vi "PI_GCS3_Sample_Application_Fault_Reaction.vi"() -> ()   [LabVIEW 2026]
doc: "This VI demonstrates how to reset a PI GCS3 system from fault axis state. The diagram shows how to combine the driver VIs for these tasks.\n\nWarning: Before running this VI, modify the interface settings on the block diagram to reflect your configuration. The predefined settings provided with the VI probably do not match your system.\n\nCompatibility: This sample requires a PI GCS 3.0 controller."
uses:
  Low Level/SpecialCommand/ModeOfOperation.ctl
  Low Level/Communication/Interface Settings.ctl
  Low Level/GeneralCommands/ParameterInfoSet.ctl
  Low Level/GeneralCommands/Status.ctl
panel:
  out "Original PID values":string[](array[string])
  out "Restored Status of motion group":T1[](array[typedef])
  out "Fault Status":T1[](array[typedef])
  out "Initial Status":T1[](array[typedef])
  out "Axis Parameter Configuration":T2[](array[typedef])
  out "error out":errorcluster
  in  "error in":errorcluster
  in  "stop":bool
  out "Identification":string
  # "This VI demonstrates how to reset a PI GCS3 system from fault axis state.\nThe diagram shows how to combine the driver VIs for these tasks. \n\nWarning: Before running this VI, modify the interface settings on the block diagram to reflect your configuration.\n                 The predefined settings provided with the VI probably do not match your system.\n\nCompatibility: This sample requires a PI GCS 3.0 controller."
  # "Error"
  # "Referenced?"
  # "Closed Loop"
  # "Axis enabled?"
  # "On target?"
  # "Fault Reaction Active?"
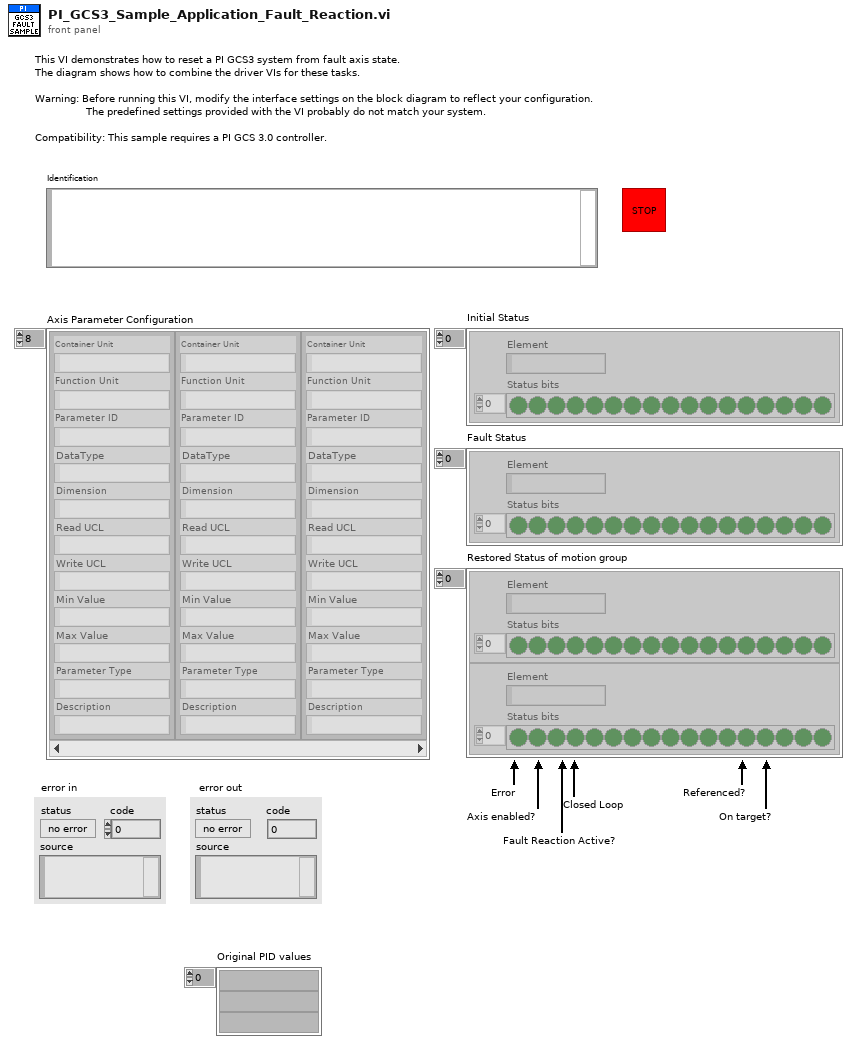
[diagram p1: front panel]
types:
  T1 = typedef "Status.ctl" = cluster{"Element":string, "Status bits":bool[]}
  T2 = typedef "ParameterInfoSet.ctl" = cluster{"Container Unit":string, "Function Unit":string, "Parameter ID":string, "DataType":string, "Dimension":string, "Read UCL":string, "Write UCL":string, "Min Value":string, "Max Value":string, "Parameter Type":string, "Description":string}
  T3 = typedef "Interface Settings.ctl" = cluster{"Interface":u16, "Timeout":u32, "RS232 settings":cluster{"Portnumber":u8, "Baudrate":u16}, "TCP/IP settings":cluster{"Host address/name":string, "Port":i32, "Board":i32, "TCP/IP Search?":bool}, "USB settings":cluster{"S/N":string, "USB Search?":bool}, "DaisyChain settings":cluster{"Register DC":bool, "DaisyChain Search?":bool, "Device ID":i32}, "DLL for Device":u16}
  T4 = typedef "ModeOfOperation.ctl" = enum16{"Open", "Open-Loop Position", "Closed-Loop Position", "Open-Loop Velocity", "Closed-Loop Velocity", "Open-Loop Force", "Closed-Loop Force", "Step Operation"}
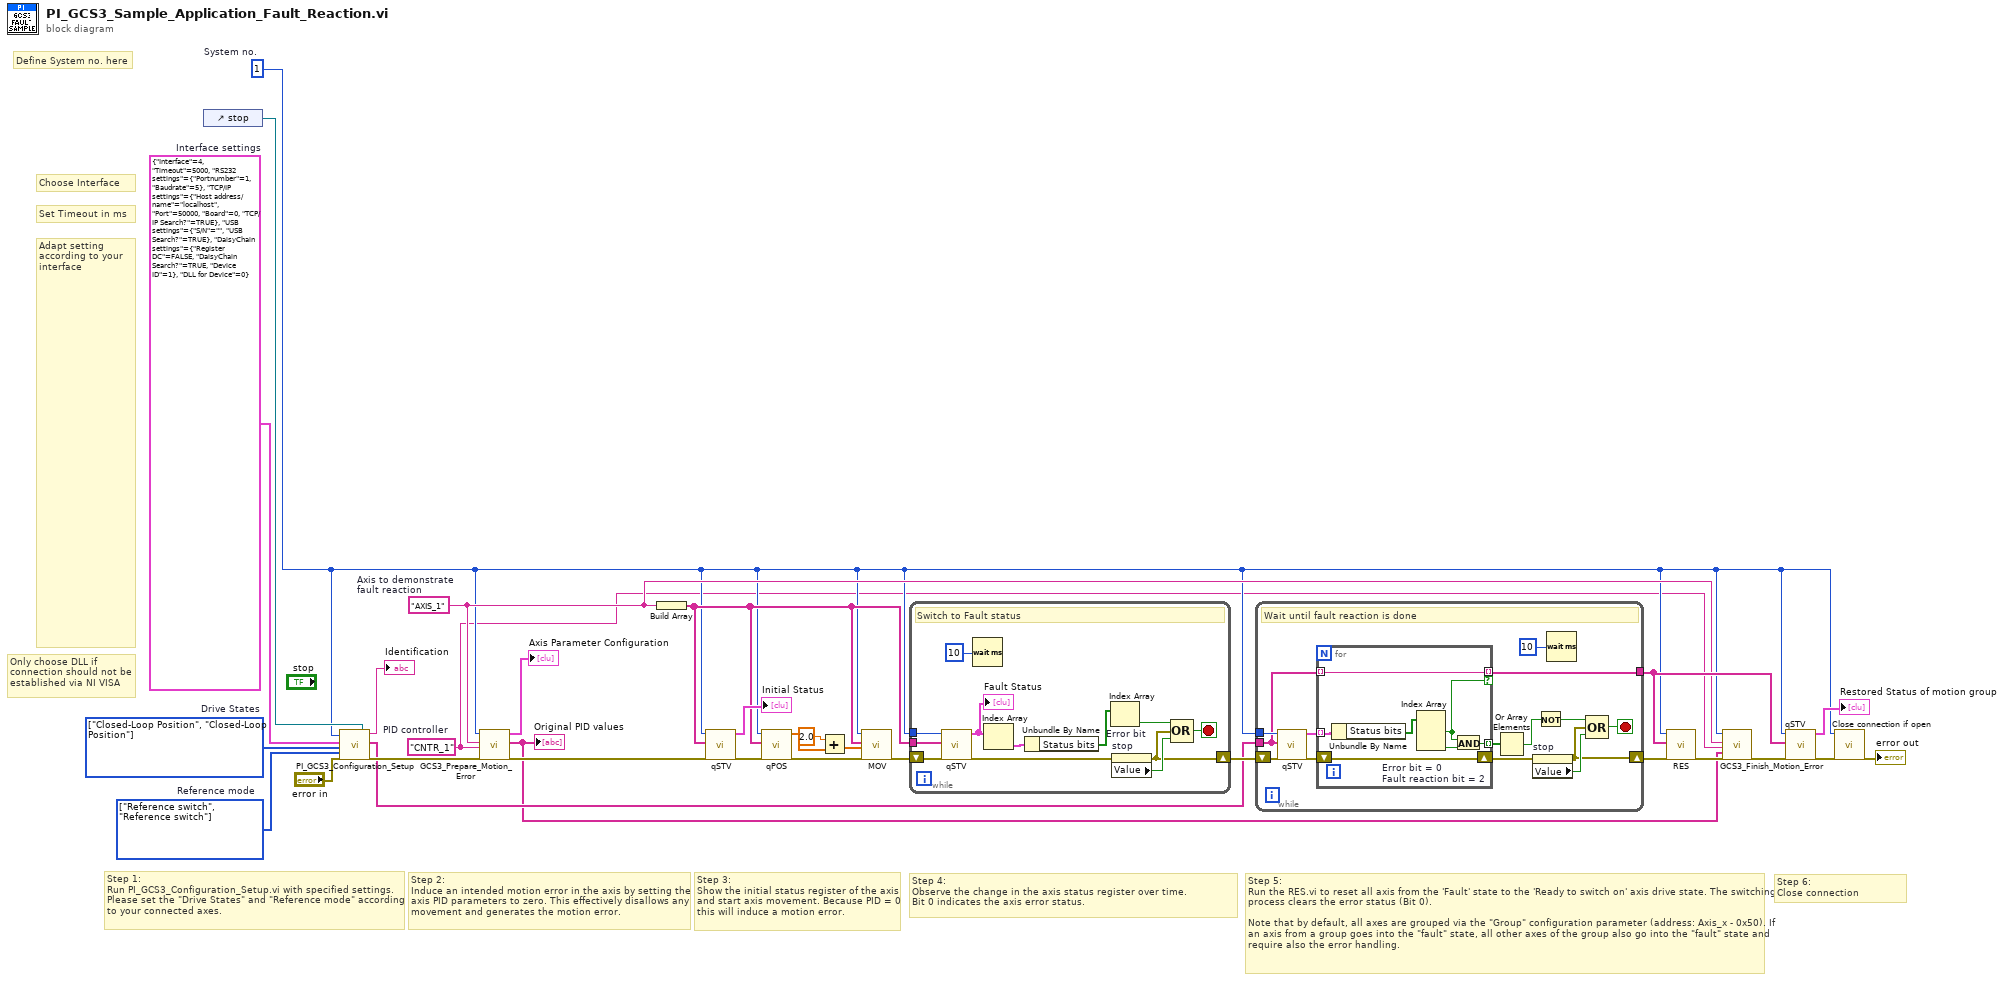
[diagram p0: block diagram]
diagram:
  w8 = T3 {"Interface"=4, "Timeout"=5000, "RS232 settings"={"Portnumber"=1, "Baudrate"=5}, "TCP/IP settings"={"Host address/name"="localhost", "Port"=50000, "Board"=0, "TCP/IP Search?"=TRUE}, "USB settings"={"S/N"="", "USB Search?"=TRUE}, "DaisyChain settings"={"Register DC"=FALSE, "DaisyChain Search?"=TRUE, "Device ID"=1}, "DLL for Device"=0}  # Interface settings
  w2 = "CNTR_1"  # PID controller
  w4 = "AXIS_1"  # Axis to demonstrate fault reaction
  w28 = T4[] [enum."Closed-Loop Position", enum."Closed-Loop Position"] items=["Open", "Open-Loop Position", "Closed-Loop Position", "Open-Loop Velocity", "Closed-Loop Velocity", "Open-Loop Force", "Closed-Loop Force", "Step Operation"]  # Drive States
  w29 = enum16{"Do not reference", "Reference switch"}[] [enum."Reference switch", enum."Reference switch"] items=["Do not reference", "Reference switch"]  # Reference mode
  w3 = 1  # System no.
  # "Define System no. here"
  # "Adapt setting according to your interface"
  # "Set Timeout in ms"
  # "Choose Interface"
  # "Only choose DLL if connection should not be established via NI VISA"
  # "Step 5:\nRun the RES.vi to reset all axis from the 'Fault' state to the 'Ready to switch on' axis drive state. The switching process clears the error status (Bit 0).\n\nNote that by default, all axes are grouped via the \"Group\" configuration parameter (address: Axis_x - 0x50). If an axis from a group goes into the \"fault\" state, all other axes of the group also go into the \"fault\" state and require also the error handling."
  # "Step 4:\nObserve the change in the axis status register over time.\nBit 0 indicates the axis error status."
  # "Step 3:\nShow the initial status register of the axis\nand start axis movement. Because PID = 0\nthis will induce a motion error."
  # "Step 2:\nInduce an intended motion error in the axis by setting the\naxis PID parameters to zero. This effectively disallows any movement and generates the motion error."
  # "Step 6:\nClose connection"
  # "Step 1:\nRun PI_GCS3_Configuration_Setup.vi with specified settings.\nPlease set the \"Drive States\" and \"Reference mode\" according\nto your connected axes."
  n1 = control-ref of="stop"() -> (w26:refnum<vi>)
  n2 = call "PI_GCS3_Configuration_Setup.vi"("System no."=w3, "Interface settings"=w8, "Mode of operation"=w28, "Reference mode"=w29, "error in"="error in", "Stop refnum"=w26) -> ("Identification"=→"Identification":string, "Conn. axis"=w11:string[], "error out"=w13:errorcluster)  [unwired: 8 in, 3 out]
  n3 = call "GCS3_Prepare_Motion_Error.vi"("System no."=w3, "Axis (ContainerUnit)"=w4, "PID controller (FunctionUnit)"=w2, "error in"=w13) -> ("Axis Parameter Configuration"=→"Axis Parameter Configuration":T2[], "Original PID values"=w1:string[], "error out"=w7:errorcluster)  [unwired: 13 in]
  "Original PID values" <- w1
  n4 = Build Array(w4) -> (w16:string[])
  n5 = call "qSTV.vi"("System no."=w3, "Status Type"=w16, "error in"=w7) -> ("Status Array"=→"Initial Status":T1[], "error out"=w20:errorcluster)  [unwired: 15 in]
  n6 = call "qPOS.vi"("System no."=w3, "Axes to query"=w16, "error in"=w20) -> ("Position"=w23:dbl[], "error out"=w24:errorcluster)  [unwired: 15 in]
  n7 = Add(x=2.0, y=w23) -> (x+y=w22:dbl[])
  n8 = call "MOV.vi"("System no."=w3, "Axes to move"=w16, "Position values"=w22, "error in"=w24) -> ("error out"=w18:errorcluster)  [unwired: 15 in]
  n9 = while {
    shift-right: [w34] -> w12
    shift-left: w18 -> [w39]
    tunnel: w3 -> [w41]
    tunnel: w16 -> [w40]
    stop <- w32 stop-if-true
    # "Switch to Fault status"
    n10 = call "qSTV.vi"("System no."=w41, "Status Type"=w40, "error in"=w39) -> ("Status Array"=w38:T1[], "error out"=w33:errorcluster)  [unwired: 15 in]
    "Fault Status" <- w38
    n11 = Wait (ms)(milliseconds to wait=u32 10) -> ()  [unwired: 1 out]
    n12 = Index Array(array=w38) -> (element=w37:T1)  [unwired: 1 in]
    n13 = Unbundle By Name(w37) -> ("Status bits"=w36:bool[])
    n14 = Index Array "Error bit"(array=w36) -> (element=w31:bool)  [unwired: 1 in]
    n15 = property on="stop" class="Bool (strict)"(error in=w33) -> (error out=w34:errorcluster, "Value"=w35:bool)  [unwired: 1 in, 1 out]
    n16 = Compound Arithmetic op=OR(w31, w34, w35) -> (w32:bool)
  }
  n17 = while {
    shift-right: [w44] -> w10
    shift-left: w12 -> [w53]
    tunnel: w11 -> [w50]
    tunnel: w3 -> [w51]
    tunnel: [w49] -> w9
    stop <- w43 stop-if-true
    # "Wait until fault reaction is done"
    n18 = call "qSTV.vi"("System no."=w51, "Status Type"=w50, "error in"=w53) -> ("Status Array"=w56:T1[], "error out"=w55:errorcluster)  [unwired: 15 in]
    n19 = for {
      tunnel: w56 -> [w63] mode=indexing
      shift-right: [w61] -> w46
      shift-left: w55 -> [w61]
      tunnel: [w59] -> w54 mode=indexing
      tunnel: w50 -> [w58] mode=indexing
      tunnel: [w58] -> w49 mode=indexing if=w57
      n20 = Unbundle By Name(w63) -> ("Status bits"=w62:bool[])
      n21 = Index Array "Error bit = 0\nFault reaction bit = 2"(array=w62) -> (element #1=w57:bool, element #3=w60:bool)  [unwired: 3 in, 1 out]
      n22 = And(x=w57, y=w60) -> (x .and. y?=w59:bool)
    }
    n23 = Or Array Elements(Boolean array=w54) -> (logical OR=w45:bool)
    n24 = property on="stop" class="Bool (strict)"(error in=w46) -> (error out=w44:errorcluster, "Value"=w47:bool)  [unwired: 1 in, 1 out]
    n25 = Not(x=w45) -> (.not. x?=w48:bool)
    n26 = Wait (ms)(milliseconds to wait=u32 10) -> ()  [unwired: 1 out]
    n27 = Compound Arithmetic op=OR(w48, w44, w47) -> (w43:bool)
  }
  n28 = call "RES.vi"("System no."=w3, "Axes to reset"=w9, "error in"=w10) -> ("error out"=w6:errorcluster)  [unwired: 16 in]
  n29 = call "GCS3_Finish_Motion_Error.vi"("System no."=w3, "Axis (ContainerUnit)"=w4, "PID controller (FunctionUnit)"=w2, "Original PID values"=w1, "error in"=w6) -> ("error out"=w5:errorcluster)  [unwired: 14 in]
  n30 = call "qSTV.vi"("System no."=w3, "Status Type"=w9, "error in"=w5) -> ("Status Array"=→"Restored Status of motion group":T1[], "error out"=w17:errorcluster)  [unwired: 15 in]
  n31 = call "Close connection if open.vi"("System no."=w3, "error in"=w17) -> ("error out"=→"error out":errorcluster)  [unwired: 16 in, 1 out]
